vi "vision 20220108 ABC.vi"(4 "error in":errorcluster) -> (0 "error out":errorcluster, 2 "index of wood":i32)   [LabVIEW 2019]
uses:
  <vilib>/vision/driver/NI_Vision_Acquisition_Software.lvlib
panel:
  out "Matches (B)":T1(array[cluster]) {"Bounding Box"."y" format="%.2f"; "Bounding Box"."x" format="%.2f"; "Position"."y" format="%.2f"; "Position"."x" format="%.2f"; "Score" format="%.2f"; "Scale" format="%.2f"; "Angle" format="%.2f"}
  out "Matches (A)":T1(array[cluster]) {"Bounding Box"."y" format="%.2f"; "Bounding Box"."x" format="%.2f"; "Position"."y" format="%.2f"; "Position"."x" format="%.2f"; "Score" format="%.2f"; "Scale" format="%.2f"; "Angle" format="%.2f"}
  out "Calibrated Matches (Pattern Matching 1)":T1(array[cluster]) {"Bounding Box"."y" format="%.2f"; "Bounding Box"."x" format="%.2f"; "Position"."y" format="%.2f"; "Position"."x" format="%.2f"; "Score" format="%.2f"; "Scale" format="%.2f"; "Angle" format="%.2f"}
  out "Image Out":T2(plugin-control)
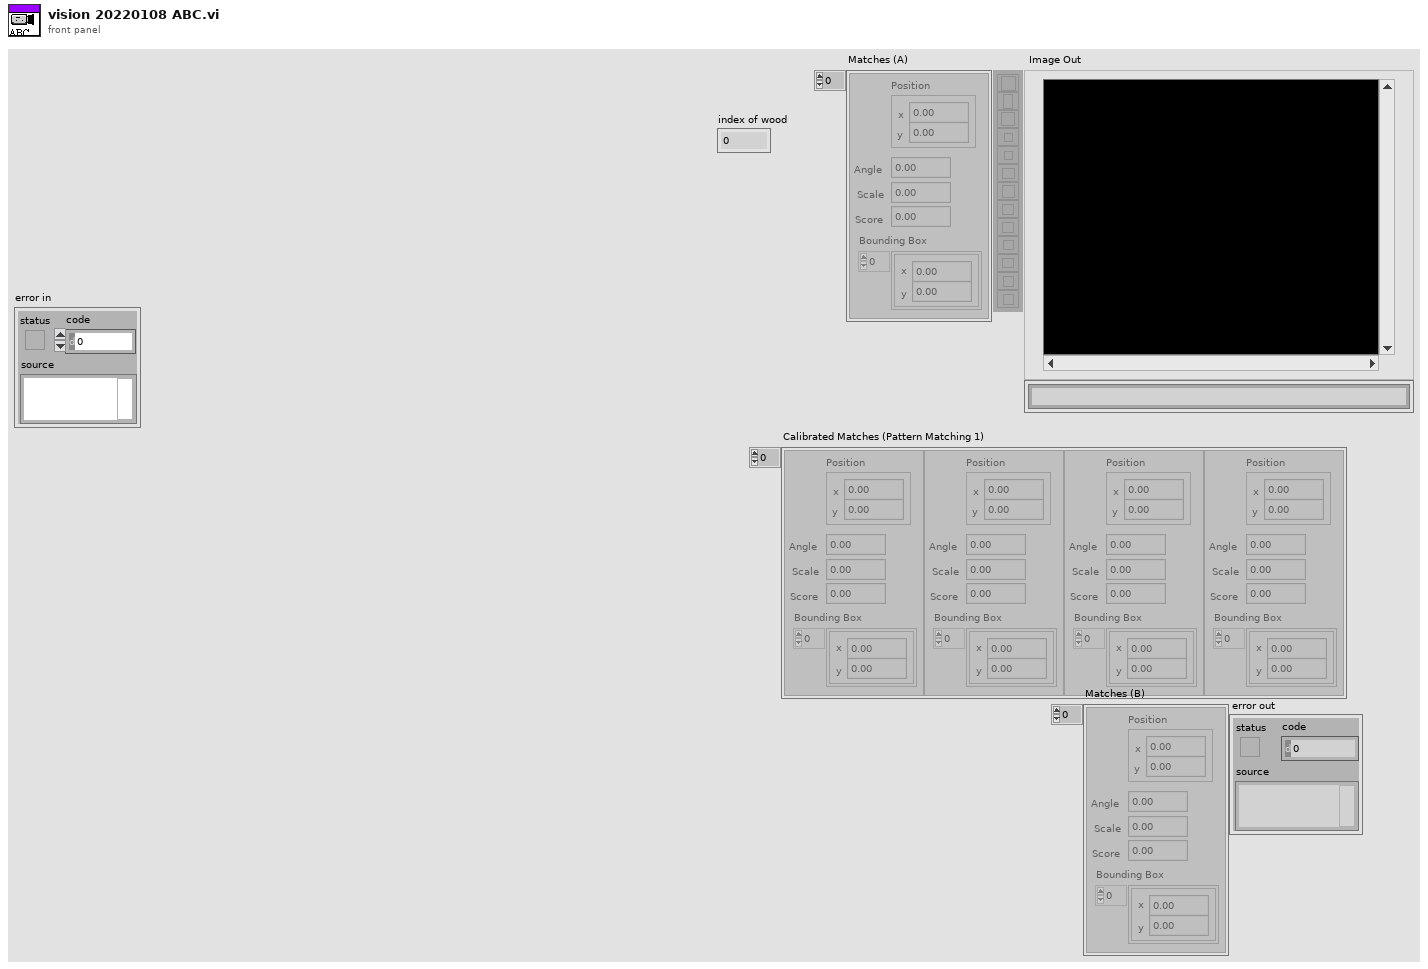
[diagram p1: front panel]
types:
  T1 = cluster{"Position":cluster{"x":sgl, "y":sgl}, "Angle":sgl, "Scale":sgl, "Score":sgl, "Bounding Box":cluster{"x":sgl, "y":sgl}[]}[]
  T2 = typedef "IMAQ Image.ctl" = refnum<image>
  T3 = typedef "IMAQdx.ctl" = refnum<k21>
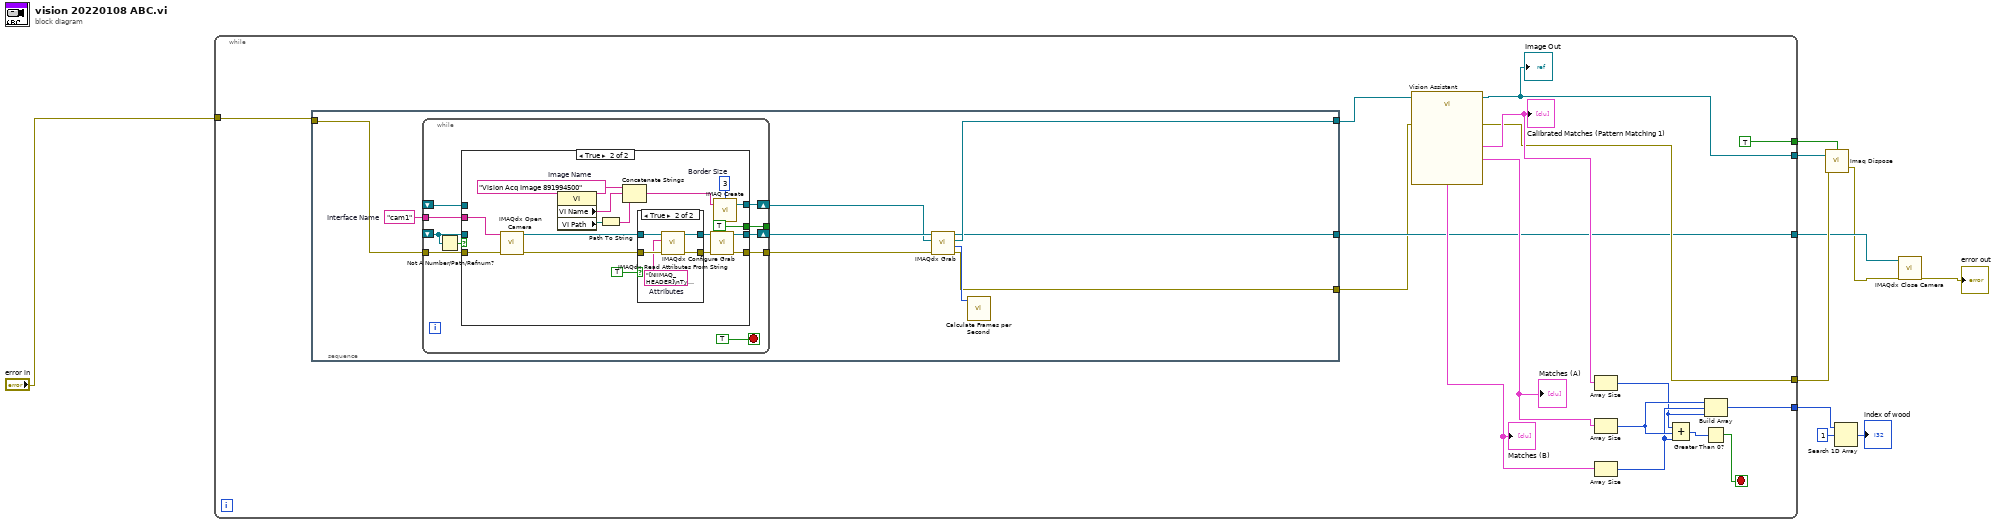
[diagram p0: block diagram]
diagram:
  n1 = while {
    tunnel: [w11] -> w10
    tunnel: "error in" -> [w18]
    tunnel: [TRUE ("All Images? (No)")] -> w6
    tunnel: [w16] -> w5
    tunnel: [w15] -> w4
    tunnel: [w14] -> w3
    stop <- w12 stop-if-true
    n2 = stacked-sequence {
      tunnel: w18 -> [w29]
      tunnel: [w32] -> w19
      tunnel: [w28] -> w13
      tunnel: [w27] -> w14
      frame #0 {
        w31 = "cam1"  # Interface Name
        n3 = while "While Loop_template0" {
          shift-right: [w45] -> w34
          shift-left: _ -> [w38]
          tunnel: [w44] -> w30
          tunnel: w29 -> [w43]
          shift-right: [w41] -> w33
          shift-left: _ -> [w40]
          tunnel: w31 -> [w39]
          tunnel: [w36] -> _
          stop <- TRUE ("_template0") stop-if-true
          n4 = Not A Number/Path/Refnum?(number/path/refnum=w38) -> (NaN/Path/Refnum?=w37:bool)
          n5 = case "Case Structure_template0" shown="True" w37 {
            tunnel: [w48 w64] -> w45
            tunnel: w38 -> [w48 _]
            tunnel: [w47 w63] -> w44
            tunnel: w43 -> [w47 w65]
            tunnel: [w46 w62] -> w41
            tunnel: w40 -> [w46 _]
            tunnel: w39 -> [_ w52]
            tunnel: [_ TRUE] -> w36
            frame False {
            }
            frame True {
              w49 = 3  # Border Size
              w57 = "Vision Acq Image 891994500"  # Image Name
              n6 = call <vilib>:"IMAQdx Open Camera.vi"("error in"=w65, "Session In"=w52) -> ("error out"=w55:errorcluster, "Session Out"=w56:T3)  [unwired: 1 in, 7 out]
              n7 = property class="VI"() -> ("VI Name"=w60:string, "VI Path"=w61:path)  [unwired: 2 in, 2 out]
              n8 = Path To String(path=w61) -> (string=w59:string)
              n9 = Concatenate Strings(w57, w60, w59) -> (w58:string)
              n10 = case shown="True" TRUE ("Init Attributes") {
                tunnel: w56 -> [w67 w72]
                tunnel: w55 -> [w66 w71]
                tunnel: [w67 w69] -> w54
                tunnel: [w66 w68] -> w53
                frame False {
                }
                frame True {
                  w70 = "[NIIMAQ_HEADER]\nType = 2\nVersion = 8\n\n[CAMERA_DATA]\nAcquisitionAttributes::Bayer::Algorithm = \"Bilinear\"\nAcquisitionAttributes::Bayer::GainB = \"1\"\nAcquisitionAttributes::Bayer::GainG = \"1\"\nAcquisitionAttributes::Bayer::GainR = \"1\"\nAcquisitionAttributes::Bayer::Pattern = \"Use hardware value\"\nAcquisitionAttributes::BitsPerPixel = \"Use hardware value\"\nAcquisitionAttributes::HardwareMaximumQueuedBufferCount = \"1000\"\nAcquisitionAttributes::HardwareRequeueBufferListThreshold = \"50\"\nAcquisitionAttributes::IgnoreFirstFrame = \"false\"\nAcquisitionAttributes::ImageDecoderCopyMode = \"Auto\"\nAcquisitionAttributes::OutputImageType = \"Auto\"\nAcquisitionAttributes::OverwriteMode = \"Get Newest\"\nAcquisitionAttributes::PixelSignedness = \"Use hardware value\"\nAcquisitionAttributes::ReceiveTimestampMode = \"None\"\nAcquisitionAttributes::ShiftPixelBits = \"false\"\nAcquisitionAttributes::SwapPixelBytes = \"false\"\nAcquisitionAttributes::Timeout = \"5000\"\nAcquisitionAttributes::VideoMode = \"160 x 120 YUY 2 30.00 fps\"\nCameraAttributes::BacklightCompensation::Mode = \"Manual\"\nCameraAttributes::BacklightCompensation::Value = \"0\"\nCameraAttributes::Brightness::Mode = \"Manual\"\nCameraAttributes::Brightness::Value = \"133\"\nCameraAttributes::Contrast::Mode = \"Manual\"\nCameraAttributes::Contrast::Value = \"5\"\nCameraAttributes::Exposure::Mode = \"AutoAperaturePriority\"\nCameraAttributes::Focus::Mode = \"Auto\"\nCameraAttributes::Pan::Mode = \"Manual\"\nCameraAttributes::Pan::Value = \"0\"\nCameraAttributes::PowerLineFrequency::Mode = \"60Hz\"\nCameraAttributes::Saturation::Mode = \"Manual\"\nCameraAttributes::Saturation::Value = \"83\"\nCameraAttributes::Sharpness::Mode = \"Manual\"\nCameraAttributes::Sharpness::Value = \"25\"\nCameraAttributes::Tilt::Mode = \"Manual\"\nCameraAttributes::Tilt::Value = \"0\"\nCameraAttributes::WhiteBalance::Mode = \"Auto\"\nCameraAttributes::Zoom::Mode = \"Manual\"\nCameraAttributes::Zoom::Value = \"0\"\n"  # Attributes
                  n11 = call <vilib>:"IMAQdx Read Attributes From String.vi"("error in"=w71, "Attributes String In"=w70, "Session In"=w72) -> ("error out"=w68:errorcluster, "Session Out"=w69:T3)  [unwired: 7 out]
                }
              }
              n12 = call <vilib>:"IMAQdx Configure Grab.vi"("error in"=w53, "Session In"=w54) -> ("error out"=w63:errorcluster, "Session Out"=w64:T3)  [unwired: 1 in, 7 out]
              n13 = call "IMAQ Create"("Border Size"=w49, "Image Name"=w58) -> ("New Image"=w62:T2)  [unwired: 2 in, 2 out]
            }
          }
        }
        n14 = call <vilib>:"IMAQdx Grab.vi"("error in"=w30, "Image In"=w33, "Session In"=w34) -> ("error out"=w28:errorcluster, "Buffer Number Out"=w35:u32, "Image Out"=w32:T2, "Session Out"=w27:T3)  [unwired: 1 in, 4 out]
        n15 = call <vilib>:"Calculate Frames per Second.vi"("Buffer Number"=w35) -> ()  [unwired: 2 in, 9 out]
      }
    }
    n16 = call "Vision Assistant"("Image In"=w19, "error in"=w13) -> ("Image Out"=w16:T2, "Matches (C)"=w26:T1, "Matches (A)"=w25:T1, "Matches (B)"=w24:T1, "error out"=w15:errorcluster)  [unwired: 21 in]
    "Image Out" <- w16
    "Calibrated Matches (Pattern Matching 1)" <- w26
    "Matches (A)" <- w25
    "Matches (B)" <- w24
    n17 = Array Size(array=w26) -> (size(s)=w20:i32)
    n18 = Array Size(array=w25) -> (size(s)=w22:i32)
    n19 = Array Size(array=w24) -> (size(s)=w21:i32)
    n20 = Compound Arithmetic op=ADD(w20, w22, w21) -> (w23:i32)
    n21 = Greater Than 0?(x=w23) -> (x > 0?=w12:bool)
    n22 = Build Array(w22, w21, w20) -> (w11:i32[])
  }
  n23 = call "Imaq Dispose"("All Images? (No)"=w6, "Image"=w5, "error in (no error)"=w4) -> ("error out"=w2:errorcluster)  [unwired: 3 in]
  n24 = Search 1D Array(1D array=w10, element=1) -> (index of element=→"index of wood":i32)  [unwired: 1 in]
  n25 = call <vilib>:"IMAQdx Close Camera.vi"("error in"=w2, "Session In"=w3) -> ("error out"=→"error out":errorcluster)  [unwired: 9 out]
